vi "OVL.vi"(0 "System no.":i32=1 min=1 max=4 step=1, 2 "Channels to set":string[](array[string]), 3 "Velocity values":dbl[](array[numeric]) format="%.6f", 4 "No.of digits":i16=4, 5 "error in":errorcluster) -> (14 "Controller error":bool, 19 "error out":errorcluster)   [LabVIEW 2020]
doc: "Sets open-loop velocity in steps/s and checks for error. Number of digits is the number of digits after the decimal point in the velocity value(s) that will be sent. Controller error is TRUE if selected system reports error code which is not 0.\n\nE-861: The velocity for open-loop stepping motion is also influenced by the step amplitude set with SSA.\nThe maximum value which can be set with OVL is given by the Open-loop velocity parameter, ID 0x7000201 (can be changed with SPA and SEP). \n\nE-870: The maximum value which can be set with OVL is given by the PIShift frequency parameter, ID 0x1F0004xx. Changing PIShift Velocity Parameter 0x1F000600 has the same effect like OVL."
panel:
  # "Sets open loop velocity in steps/s and checks for error."
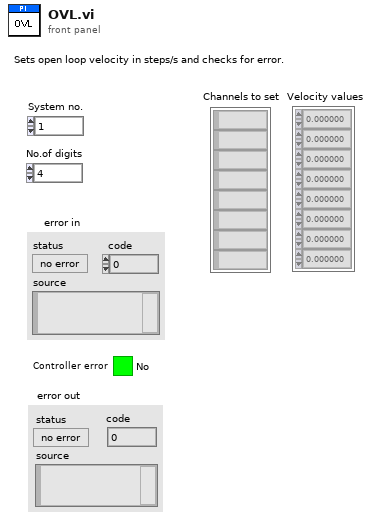
[diagram p1: front panel]
types:
  T1 = enum16{"Disable error check", "Force error check", "Use global settings"}
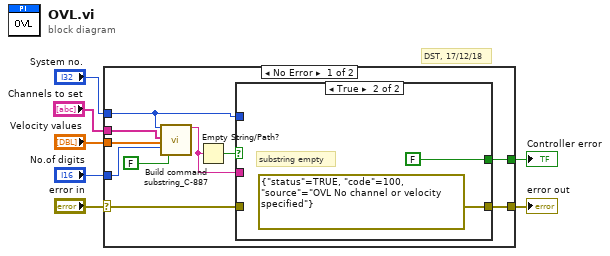
[diagram p0: block diagram]
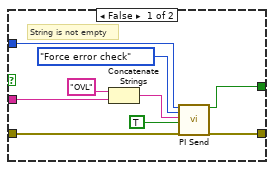
[diagram p2: hidden frame]
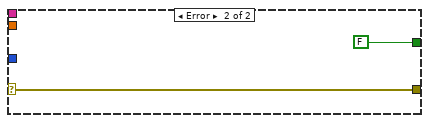
[diagram p3: hidden frame]
diagram:
  # "DST, 17/12/18"
  n1 = case shown="No Error" "error in" {
    selector: "error in" -> [w11 w30]
    tunnel: [w17 w30] -> w7
    tunnel: "Velocity values" -> [w16 _]
    tunnel: "No.of digits" -> [w15 _]
    tunnel: "System no." -> [w13 _]
    tunnel: "Channels to set" -> [w14 _]
    tunnel: [w8 FALSE ("Controller error")] -> w1
    frame No Error {
      n2 = call "Build command substring_C-887.vi"("System no."=w13, "Affected axes"=w14, "Parameters"=w16, "No. of digits"=w15, "Parameter no. format \n(Decimal: FALSE)"=FALSE ("Parameter no. format \n(Decimal: FALSE)")) -> ("Command substring"=w10:string)  [unwired: 2 in, 12 out]
      n3 = Empty String/Path?(string/path=w10) -> (empty?=w9:bool)
      n4 = case shown="True" w9 {
        tunnel: w10 -> [w25 _]
        tunnel: [w19 errorcluster {"status"=TRUE, "code"=100, "source"="OVL No channel or velocity specified"} ("error out")] -> w17
        tunnel: w11 -> [w22 _]
        tunnel: w13 -> [w21 _]
        tunnel: [w20 FALSE ("Controller error")] -> w8
        frame False {
          # "String is not empty"
          n5 = Concatenate Strings("OVL", w25) -> (w23:string)
          n6 = call "PI Send.vi"("System no."=w21, "Error check settings"=T1."Force error check", "String to send"=w23, "Attach termination char.?"=TRUE ("Attach Linefeed?"), "error in"=w22) -> ("Controller error"=w20:bool, "error out"=w19:errorcluster)  [unwired: 1 in, 12 out]
        }
        frame True {
          # "substring empty"
        }
      }
    }
    frame Error {
    }
  }
  "error out" <- w7
  "Controller error" <- w1
